vi "Record.vi"() -> ()   [LabVIEW 2019]
uses:
  <vilib>/DAQmx/read.llb/DAQmx Read (Analog 1D Wfm NChan NSamp).vi
  <vilib>/DAQmx/create/channels.llb/DAQmx Create Channel (AI-Voltage-Basic).vi
  <vilib>/DAQmx/configure/timing.llb/DAQmx Timing (Sample Clock).vi
  <vilib>/DAQmx/miscellaneous.llb/DAQmx Fill In Error Info.vi
panel:
  out "Elapsed Time (s)":dbl
  in  "Record":bool
  out "Waveform Graph":waveform(dbl)[](graph)
  in  "stop":bool
  in  "file path":path
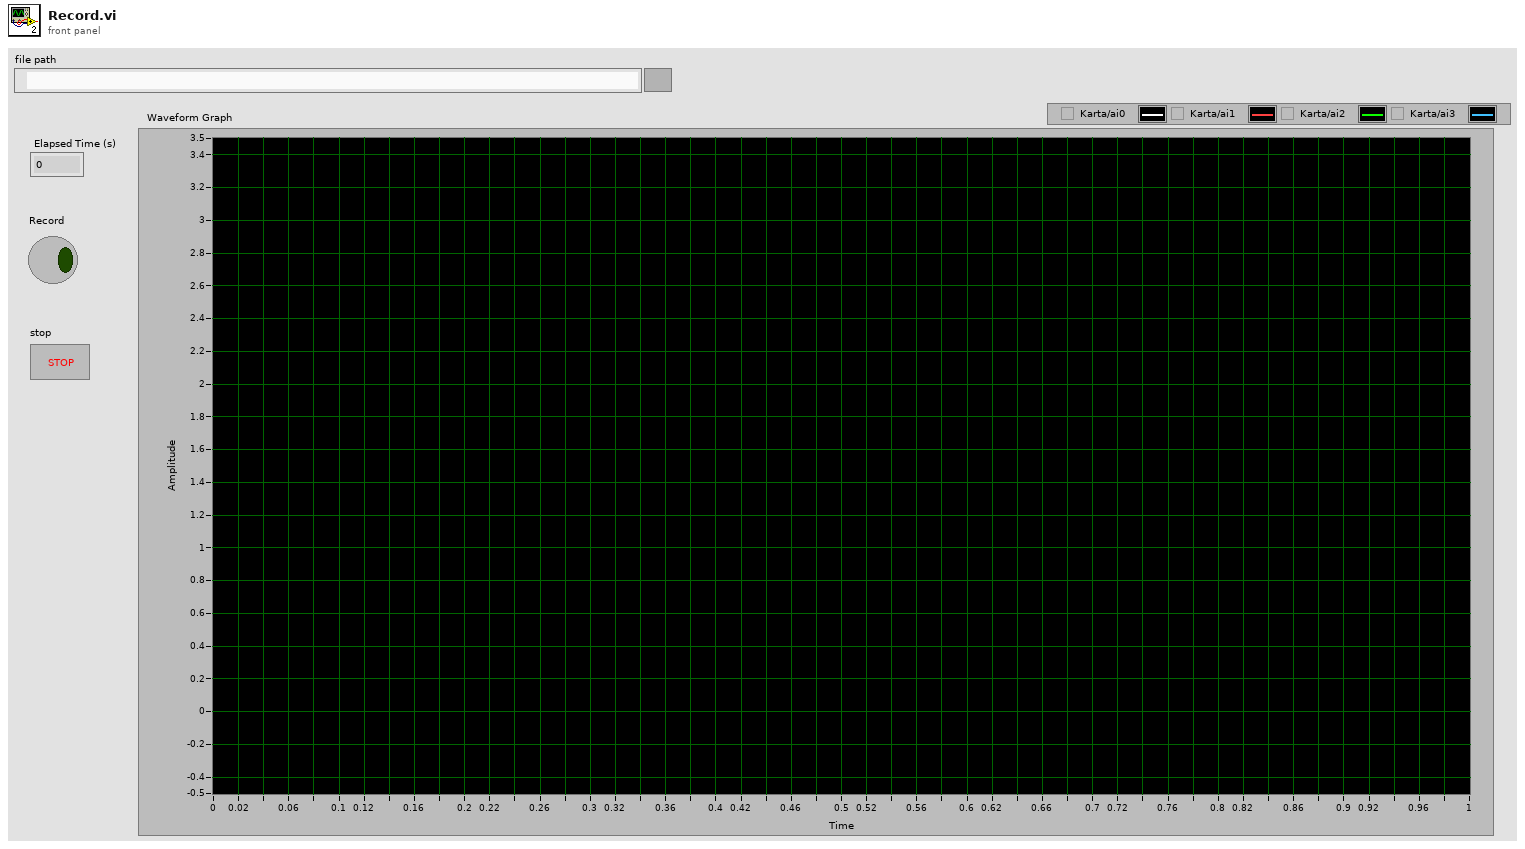
[diagram p1: front panel]
types:
  T1 = enum16{"open", "open or create", "create or replace", "create", "open (read-only)"}
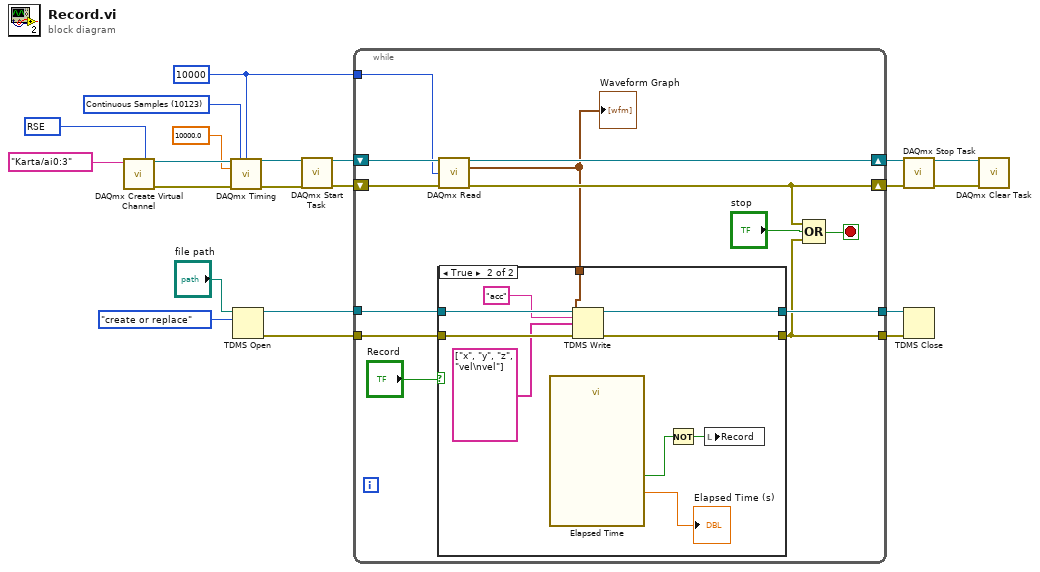
[diagram p0: block diagram]
diagram:
  w1 = 10083 items=["Default"=-1, "RSE"=10083, "NRSE"=10078, "Differential"=10106, "Pseudodifferential"=12529] ("input terminal configuration")
  w4 = 10000 ("samples per channel")
  w9 = 10123 items=["Finite Samples"=10178, "Continuous Samples"=10123, "Hardware Timed Single Point"=12522] ("sample mode")
  n1 = call-poly <vilib>:"DAQmx Create Virtual Channel.vi"("input terminal configuration"=w1, "physical channels"=tag "Karta/ai0:3") -> ("task out"=w21:refnum<k21>, "error out"=w20:errorcluster)  [unwired: 12 in]
  n2 = call-poly <vilib>:"DAQmx Timing.vi"("task/channels in"=w21, "sample mode"=w9, "samples per channel"=w4, "rate"=10000.0, "error in"=w20) -> ("task out"=w19:refnum<k21>, "error out"=w18:errorcluster)  [unwired: 9 in]
  n3 = TDMS Open(10:T1."create or replace" ("operation (0:open)"), 11:"file path") -> (0:w7:errorcluster, 3:w8:refnum<k34>)  [unwired: 5 in]
  n4 = call <vilib>:"DAQmx Start Task.vi"("task/channels in"=w19, "error in"=w18) -> ("task out"=w17:refnum<k21>, "error out"=w16:errorcluster)  [unwired: 12 in]
  n5 = while {
    tunnel: w8 -> [w30]
    tunnel: w7 -> [w31]
    tunnel: [w29] -> w6
    tunnel: [w26] -> w5
    tunnel: w4 -> [w28]
    shift-right: [w32] -> w15
    shift-left: w17 -> [w34]
    shift-right: [w25] -> w14
    shift-left: w16 -> [w33]
    stop <- w27 stop-if-true
    n6 = call-poly <vilib>:"DAQmx Read.vi"("task/channels in"=w34, "number of samples per channel"=w28, "error in"=w33) -> ("task out"=w32:refnum<k21>, "data"=w23:waveform(dbl)[], "error out"=w25:errorcluster)  [unwired: 10 in]
    "Waveform Graph" <- w23
    n7 = case shown="True" "Record" {
      tunnel: w31 -> [w35 w46]
      tunnel: w30 -> [w36 w45]
      tunnel: [w36 w44] -> w29
      tunnel: [w35 w41] -> w26
      tunnel: w23 -> [_ w40]
      frame False {
      }
      frame True {
        n8 = call "Elapsed Time"() -> ("Elapsed Time (s)"=→"Elapsed Time (s)":dbl, "Time has Elapsed"=w38:bool)  [unwired: 12 in, 6 out]
        n9 = TDMS Write(0:w45, 5:"acc" ("group name in (Untitled)"), 7:string[] ["x", "y", "z", "vel\nvel"] ("channel name(s) in (Untitled)"), 9:w40, 11:w46) -> (4:w44:refnum<k34>, 15:w41:errorcluster)  [unwired: 1 in, 2 out]
        n10 = Not(x=w38) -> (.not. x?=w37:bool)
        n11 = local write "Record"(w37) -> ()
      }
    }
    n12 = Compound Arithmetic op=OR(w25, "stop", w26) -> (w27:bool)
  }
  n13 = call <vilib>:"DAQmx Stop Task.vi"("task/channels in"=w15, "error in"=w14) -> ("task out"=w13:refnum<k21>, "error out"=w12:errorcluster)  [unwired: 12 in]
  n14 = TDMS Close(8:w5, 11:w6) -> ()  [unwired: 2 out]
  n15 = call <vilib>:"DAQmx Clear Task.vi"("task in"=w13, "error in"=w12) -> ()  [unwired: 13 in, 1 out]
